vi "Decode PNG Palette Chunk.vi"(10 "error in (no error)":errorcluster, 11 "data":u8[](array[numeric])) -> (2 "error out":errorcluster, 3 "Colors":u32[](array[colorbox]))   [LabVIEW 2021, in "Files.lvlib"]
uses:
  Files.lvlib
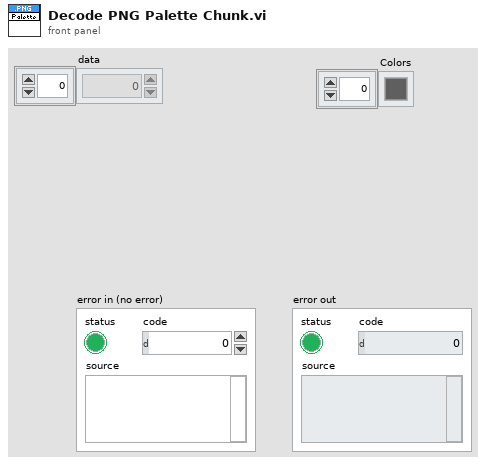
[diagram p1: front panel]
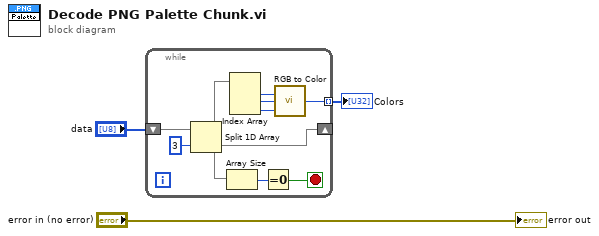
[diagram p0: block diagram]
diagram:
  n1 = while {
    shift-right: [w11] -> _
    shift-left: "data" -> [w13]
    tunnel: [w4] -> w1 mode=indexing
    stop <- w9 stop-if-true
    n2 = Split 1D Array(array=w13, index=3) -> (first subarray=w8:u8[], second subarray=w11:u8[])
    n3 = Array Size(array=w11) -> (size(s)=w10:i32)
    n4 = Index Array(array=w8) -> (element #1=w7:u8, element #2=w6:u8, element #3=w5:u8)  [unwired: 3 in]
    n5 = Equal To 0?(x=w10) -> (x = 0?=w9:bool)
    n6 = call <vilib>:"RGB to Color.vi"("B"=w5, "G"=w6, "R"=w7) -> ("Color"=w4:u32)
  }
  "Colors" <- w1
  "error out" <- "error in (no error)"
